vi "火焰删除.vi"(8 "error in (no error)":errorcluster, 9 "Image dst":T1, 11 "Image source":T1) -> (0 "error out":errorcluster, 3 "Threshold Image":T1(plugin-control))   [LabVIEW 2018]
uses:
  <vilib>/vision/Image Controls.llb/IMAQ Image.ctl
  <vilib>/vision/NI_Vision_Development_Module.lvlib
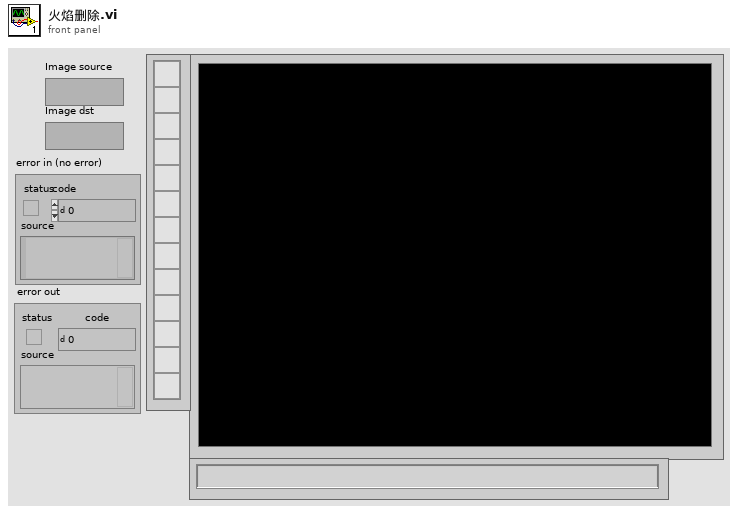
[diagram p1: front panel]
types:
  T1 = typedef "IMAQ Image.ctl" = refnum<image>
  T2 = typedef "Image Type" = u32
  T3 = cluster{"X Size":i32, "Y Size":i32, "% Tolerance":i32}
  T4 = typedef "ROI Descriptor" = cluster{"Global Rectangle":i32[], "Contours":cluster{"ID":enum32{"External", "Internal"}, "Type":u32, "Coordinates":i32[]}[]}
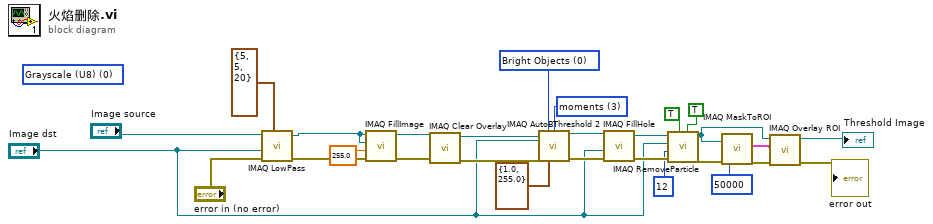
[diagram p0: block diagram]
diagram:
  (unwired) T2 0 items=["Grayscale (U8)", "Grayscale (I16)", "Grayscale (SGL)", "Complex (CSG)", "RGB (U32)", "HSL (U32)", "RGB (U64)", "Grayscale (U16)"] ("Image Type")
  w23 = u32 0 items=["Bright Objects", "Dark Objects"] ("Look For (Bright Objects)")
  w25 = 3 items=["clustering", "entropy", "metric", "moments", "inter-class variance"] ("Method")
  n1 = call "IMAQ LowPass"("Image Src"="Image source", "Size & Tolerance"=T3 {"X Size"=5, "Y Size"=5, "% Tolerance"=20}, "Image Dst"="Image dst", "error in (no error)"="error in (no error)") -> ("Image Dst Out"=w26:T1, "error out"=w8:errorcluster)  [unwired: 3 in]
  n2 = call "IMAQ FillImage"("error in (no error)"=w8, "Pixel Value (U8, U16, I16, Float)"=sgl 255.0, "Image Mask"=w26, "Image"=w26) -> ("error out"=w4:errorcluster, "Image Out"=w6:T1)  [unwired: 6 in]
  n3 = call "IMAQ Clear Overlay"("error in (no error)"=w4, "Image"=w6) -> ("error out"=w3:errorcluster, "Image Out"=w5:T1)  [unwired: 8 in]
  n4 = call "IMAQ AutoBThreshold 2"("Image Src"=w5, "Look For (Bright Objects)"=w23, "Method (clustering)"=w25, "Image Dst"="Image dst", "error in (no error)"=w3, "Threshold Limits"=cluster{"Lower value":sgl, "Upper value":sgl} {"Lower value"=1.0, "Upper value"=255.0}) -> ("Image Dst Out"=w11:T1, "error out"=w24:errorcluster)  [unwired: 2 in, 6 out]
  n5 = call "IMAQ FillHole"("error in (no error)"=w24, "Image Dst"="Image dst", "Image Src"=w11) -> ("error out"=w20:errorcluster, "Image Dst Out"=w21:T1)  [unwired: 3 in]
  n6 = call "IMAQ RemoveParticle"("Connectivity 4/8 (8)"=TRUE, "Square/Hexa (Square)"=TRUE, "error in (no error)"=w20, "Number of Erosion"=12, "Image Dst"="Image dst", "Image Src"=w21) -> ("error out"=w16:errorcluster, "Image Dst Out"=w14:T1)  [unwired: 4 in]
  n7 = call "IMAQ MaskToROI"("Image"=w14, "Max number of vectors in ROI"=50000, "error in (no error)"=w16) -> ("ROI Descriptor"=w15:T4, "error out"=w13:errorcluster)  [unwired: 4 in, 1 out]
  n8 = call "IMAQ Overlay ROI"("error in (no error)"=w13, "ROI Descriptor"=w15, "Image"=w14) -> ("error out"=→"error out":errorcluster, "Image Out"=→"Threshold Image":T1)  [unwired: 7 in]
